vi "Insert Left SubPanel.vi"(8 "error in (no error)":errorcluster, 9 "ActorQName":string, 10 "ActorVI Ref":refnum<vi>, 11 "UI_Left_Right in":refnum<class "UI_Left_Right.lvclass">) -> (0 "error out":errorcluster, 3 "UI_Left_Right out":refnum<class "UI_Left_Right.lvclass">)   [LabVIEW 2021, in "UI_Left_Right.lvclass"]
uses:
  UI_Left_Right.lvclass
  C:/Program Files (x86)/National Instruments/LabVIEW 2021/vi.lib/ActorFramework/Actor/Actor.lvclass
  <vilib>/ActorFramework/Actor/Actor.lvclass/Actor.ctl
  UI_Left_Right.lvclass/UI_Left_Right.ctl
  <vilib>/ActorFramework/Message Enqueuer/Message Enqueuer.lvclass/Message Enqueuer.ctl
  <vilib>/ActorFramework/Message Enqueuer/Enqueue.vi
  <userlib>/John_Lib/AbstractActorTemplate/UIActorTop Messages/UI Initialize Msg/UI Initialize Msg.lvclass
  C:/Program Files (x86)/National Instruments/LabVIEW 2021/vi.lib/ActorFramework/Message/Message.lvclass
  <vilib>/ActorFramework/Message Priority Queue/Priority Enqueue.vi
  <vilib>/ActorFramework/Actor/Actor.lvclass
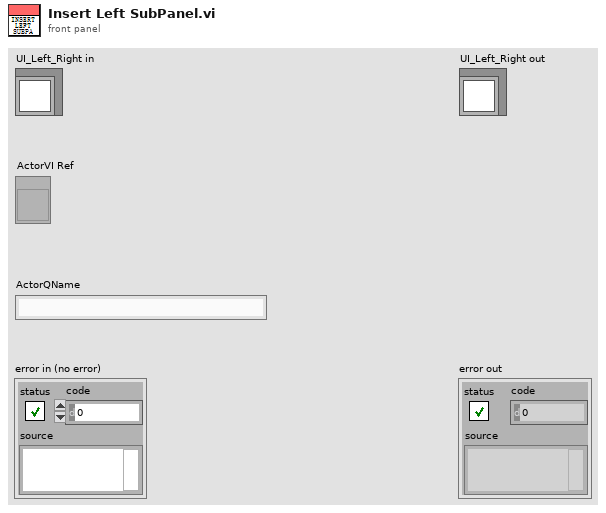
[diagram p1: front panel]
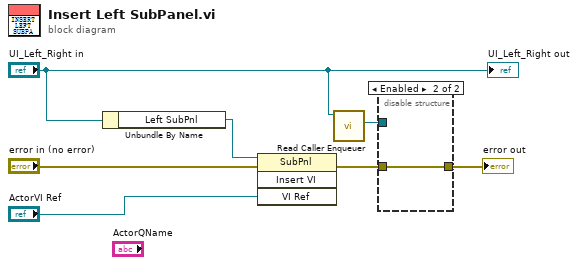
[diagram p0: block diagram]
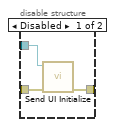
[diagram p2: hidden frame]
diagram:
  n1 = Unbundle By Name("UI_Left_Right in") -> ("Left SubPnl"=w7:refnum<vi>)
  n2 = invoke class="SubPnl" method="Insert VI"(reference=w7, error in="error in (no error)", "VI Ref"="ActorVI Ref") -> (error out=w2:errorcluster)  [unwired: 1 in, 3 out]
  n3 = call <vilib>:"Read Caller Enqueuer.vi"("Actor"="UI_Left_Right in") -> ("Caller Enqueuer"=w4:refnum<class "Message Enqueuer.lvclass">)  [unwired: 10 in]
  n4 = disable-structure shown="Enabled" {
    disable-tunnel: w4 -> [w10 _]
    disable-tunnel: w2 -> [w9 w11]
    disable-tunnel: [w8 w11] -> w1
    frame Disabled {
      n5 = call <userlib>:"Send UI Initialize.vi"("error in (no error)"=w9, "Message Enqueuer"=w10) -> ("error out"=w8:errorcluster)  [unwired: 8 in, 1 out]
    }
    frame Enabled {
    }
  }
  "error out" <- w1
  "UI_Left_Right out" <- "UI_Left_Right in"
